vi "no_apper.vi"(1 "String":string="C", 2 "Array":cluster{string, "number of columns":i32}[](array[cluster])) -> (0 "Numeric":i32)   [LabVIEW 2019]
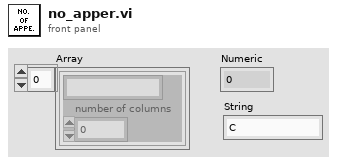
[diagram p1: front panel]
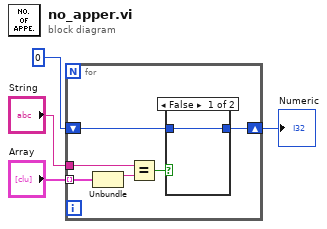
[diagram p0: block diagram]
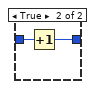
[diagram p2: hidden frame]
diagram:
  n1 = for {
    tunnel: "Array" -> [w9] mode=indexing
    shift-right: [w7] -> w4
    shift-left: 0 -> [w8]
    tunnel: "String" -> [w5]
    n2 = Unbundle(w9) -> (w10:string)  [unwired: 1 out]
    n3 = Equal?(x=w5, y=w10) -> (x = y?=w6:bool)
    n4 = case shown="False" w6 {
      tunnel: w8 -> [w11 w13]
      tunnel: [w11 w12] -> w7
      frame False {
      }
      frame True {
        n5 = Increment(x=w13) -> (x+1=w12:i32)
      }
    }
  }
  "Numeric" <- w4
